vi "Station Display Instrument Info.vi"(8 "error in (no error)":errorcluster, 11 "Station in":refnum<class "Station.lvclass">) -> (0 "error out":errorcluster, 2 "Table Control":string[][](table), 3 "Station out":refnum<class "Station.lvclass">)   [LabVIEW 2018, in "Station.lvclass"]
uses:
  Station.lvclass
  <vilib>/Utility/file.llb/Read Delimited Spreadsheet (string).vi
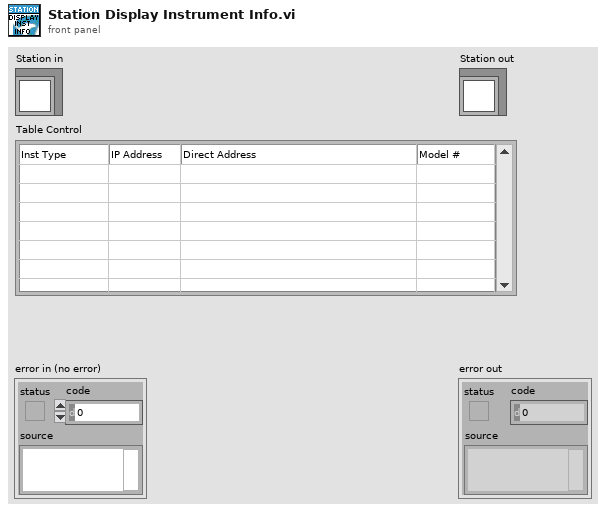
[diagram p1: front panel]
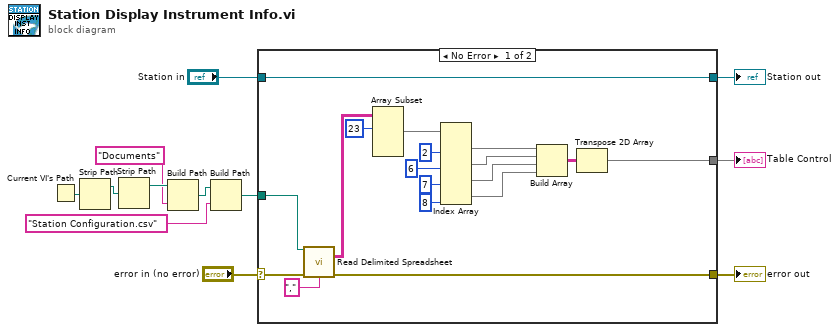
[diagram p0: block diagram]
diagram:
  n1 = Current VI's Path() -> (path=w6:path)
  n2 = Strip Path(path=w6) -> (stripped path=w7:path)  [unwired: 1 out]
  n3 = Strip Path(path=w7) -> (stripped path=w12:path)  [unwired: 1 out]
  n4 = Build Path(base path=w12, name or relative path="Documents") -> (appended path=w10:path)
  n5 = Build Path(base path=w10, name or relative path="Station Configuration.csv") -> (appended path=w8:path)
  n6 = case shown="No Error" "error in (no error)" {
    selector: "error in (no error)" -> [w30 w32]
    tunnel: [w28 w32] -> w3
    tunnel: w8 -> [w29 _]
    tunnel: [w16 _] -> w5
    tunnel: "Station in" -> [w13 w31]
    tunnel: [w13 w31] -> w1
    frame No Error {
      n7 = call-poly <vilib>:"Read Delimited Spreadsheet.vi"("file path (dialog if empty)"=w29, "error in (no error)"=w30, "delimiter (\\t)"="," ("delimiter (\\t)")) -> ("all rows"=w26:string[][], "error out"=w28:errorcluster)  [unwired: 7 in, 4 out]
      n8 = Array Subset(array=w26, index (row)=23 ("index")) -> (w24:string[][])  [unwired: 3 in]
      n9 = Index Array(array=w24, index (col) #1=2 ("disabled index (col)"), index (col) #2=6 ("index (col)"), index (col) #3=7 ("index (col)"), index (col) #4=8 ("index (col)")) -> (element #1=w20:string[], element #2=w19:string[], element #3=w18:string[], element #4=w14:string[])  [unwired: 4 in]
      n10 = Build Array(w20, w19, w18, w14) -> (w17:string[][])
      n11 = Transpose 2D Array(2D array=w17) -> (transposed array=w16:string[][])
    }
    frame Error {
    }
  }
  "error out" <- w3
  "Station out" <- w1
  "Table Control" <- w5
